vi "comp.vi"(10 "expression régulière":string, 11 "strout":string) -> (3 "Boolean":bool)   [LabVIEW 2020]
uses:
  <vilib>/regexp/Match Regular Expression.xnode
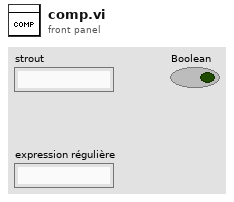
[diagram p1: front panel]
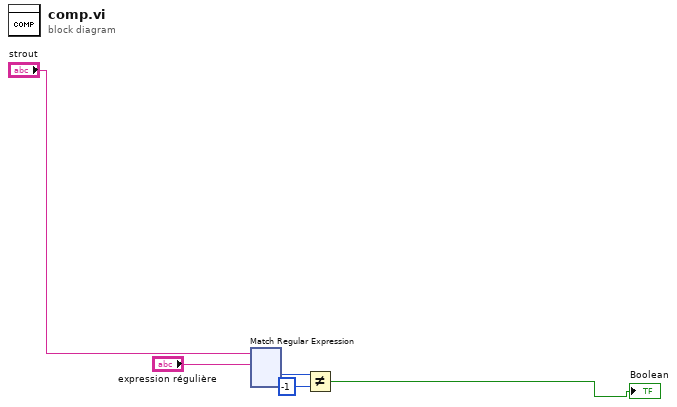
[diagram p0: block diagram]
diagram:
  n1 = xnode "Match Regular Expression"("chaîne en entrée"="strout", "expression régulière"="expression régulière") -> ("offset après correspondance"=w1:i32)  [unwired: 4 in, 4 out]
  n2 = Not Equal? ("Différents ?")(x=w1, y=-1) -> (x != y?=→"Boolean":bool)
